vi "Result to Data Warehouse Package.vi"(6 "File Data Objs":T1[](array[typedef]), 7 "Temp Folder":path, 8 "error in":errorcluster, 9 "Test Result":T2={"#attributes"={"Version"="MTE_1.0.0"}, "Station"={"Name"="", "PN"="", "SN"="", "Rev"="", "PC Name"="", "Location"="", "HW_Config"={"HW_Item"=[]}, "SW_Config"={"SW_Item"=[]}}, "Test Run"={"Operator"="", "Start Time"=timestamp(0 s since 1904-01-01), "Duration(s)"=0.0, "Mode"="", "Comment"="", "ProcessStep"=""}, "Test Sequence"={"Name"="", "Config"={"Config_Item"=[]}}, "UUTs"={"UUT"=[]}} {"UUTs"."UUT"."Measurements"."Measurement"."Status" items=["LOG", "PASS", "FAIL", "ERROR"]}, 10 "File Name":string, 11 "Folder":path) -> (0 "error out":errorcluster)   [LabVIEW 2018]
uses:
  TestResult.FullResultData.ctl
  TestResult.Station Info.ctl
  TestResult.HW Item.ctl
  TestResult.SW Item.ctl
  TestResult.Test Run Info.ctl
  TestResult.Test Info.ctl
  TestResult.UUT Result.ctl
  TestResult.Symptom.ctl
  TestResult.Symptom.State.ctl
  Result.Measurement Item.ctl
  Result.Measurement and Attribute Item Status.ctl
  TestResult.UUTInfo.ctl
  Reports/Report.Result FileDataObject.ctl
  <vilib>/KATE/Files/File Utils.lvlib
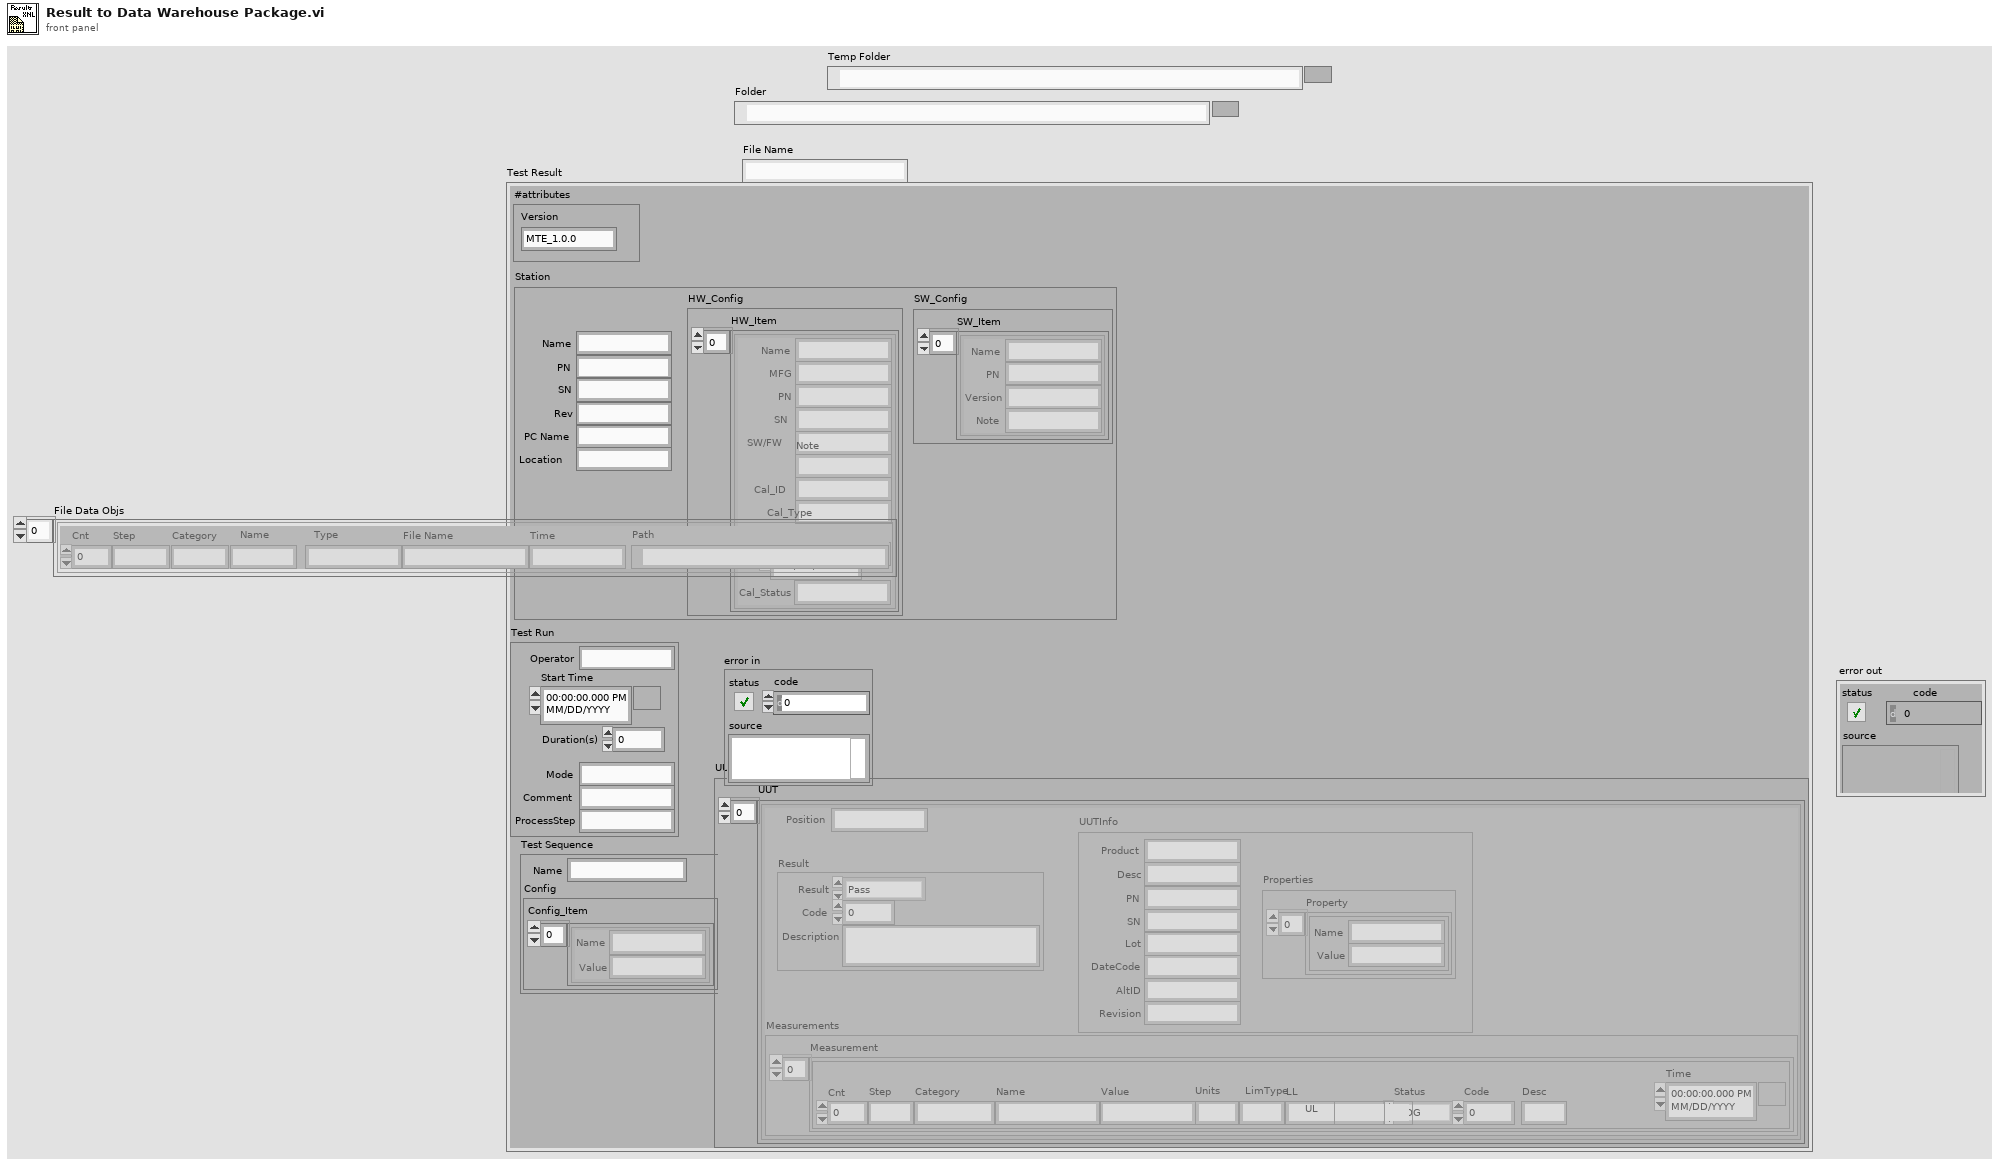
[diagram p1: front panel]
types:
  T1 = typedef "Report.Result FileDataObject.ctl" = cluster{"Cnt":i32, "Step":string, "Category":string, "Name":string, "Type":string, "File Name":string, "Time":string, "Path":path}
  T2 = typedef "TestResult.FullResultData.ctl" = cluster{"#attributes":cluster{"Version":string}, "Station":T3, "Test Run":T6, "Test Sequence":T7, "UUTs":cluster{"UUT":T8[]}}
  T3 = typedef "TestResult.Station Info.ctl" = cluster{"Name":string, "PN":string, "SN":string, "Rev":string, "PC Name":string, "Location":string, "HW_Config":cluster{"HW_Item":T4[]}, "SW_Config":cluster{"SW_Item":T5[]}}
  T4 = typedef "TestResult.HW Item.ctl" = cluster{"Name":string, "MFG":string, "PN":string, "SN":string, "SW/FW":string, "Note":string, "Cal_ID":string, "Cal_Type":string, "Cal_Due_Date":timestamp, "Cal_Status":string}
  T5 = typedef "TestResult.SW Item.ctl" = cluster{"Name":string, "PN":string, "Version":string, "Note":string}
  T6 = typedef "TestResult.Test Run Info.ctl" = cluster{"Operator":string, "Start Time":timestamp, "Duration(s)":dbl, "Mode":string, "Comment":string, "ProcessStep":string}
  T7 = typedef "TestResult.Test Info.ctl" = cluster{"Name":string, "Config":cluster{"Config_Item":cluster{"Name":string, "Value":string}[]}}
  T8 = typedef "TestResult.UUT Result.ctl" = cluster{"Position":string, "Result":T9, "Measurements":cluster{"Measurement":T11[]}, "UUTInfo":T13}
  T9 = typedef "TestResult.Symptom.ctl" = cluster{"Result":T10, "Code":i32, "Description":string}
  T10 = typedef "TestResult.Symptom.State.ctl" = enum16{"Pass", "Fail", "Error", "Aborted", "Completed", "Logged"}
  T11 = typedef "Result.Measurement Item.ctl" = cluster{"Cnt":i32, "Step":string, "Category":string, "Name":string, "Value":string, "Units":string, "LimType":string, "LL":string, "UL":string, "Status":T12, "Code":i32, "Desc":string, "Time":timestamp}
  T12 = typedef "Result.Measurement and Attribute Item Status.ctl" = i32
  T13 = typedef "TestResult.UUTInfo.ctl" = cluster{"Product":string, "Desc":string, "PN":string, "SN":string, "Lot":string, "DateCode":string, "AltID":string, "Revision":string, "Properties":cluster{"Property":cluster{"Name":string, "Value":string}[]}}
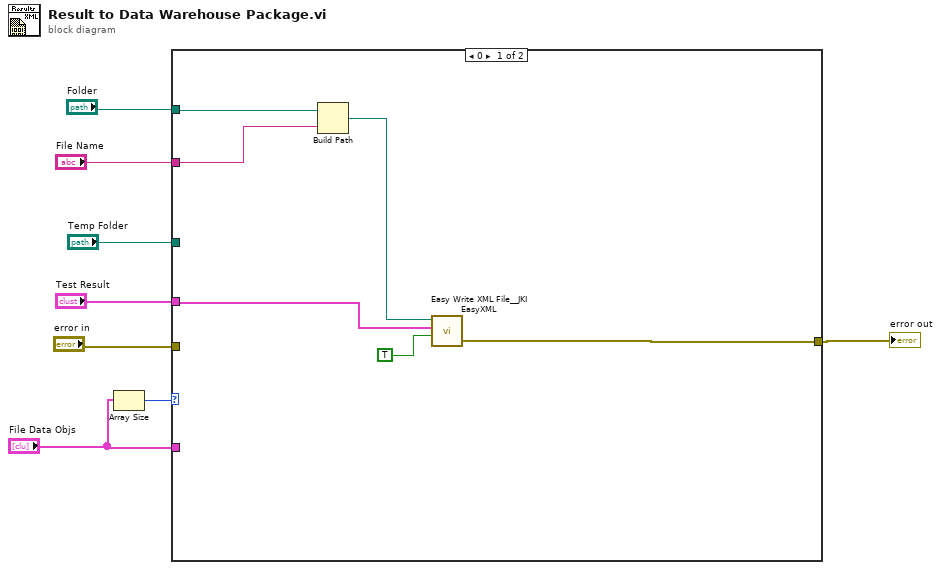
[diagram p0: block diagram]
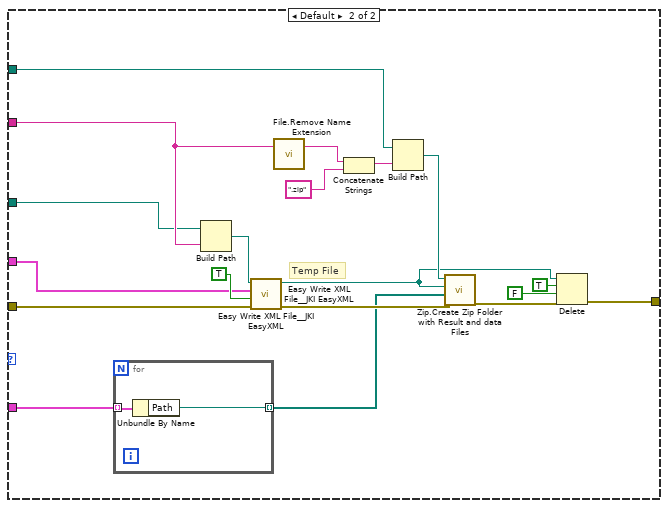
[diagram p2: hidden frame]
diagram:
  n1 = Array Size(array="File Data Objs") -> (size(s)=w2:i32)
  n2 = case shown="0" w2 {
    tunnel: "Test Result" -> [w12 w18]
    tunnel: "error in" -> [_ w33]
    tunnel: "File Data Objs" -> [_ w16]
    tunnel: "File Name" -> [w13 w30]
    tunnel: "Folder" -> [w14 w27]
    tunnel: [w10 w23] -> w4
    tunnel: "Temp Folder" -> [_ w17]
    frame 0 {
      n3 = Build Path(base path=w14, name or relative path=w13) -> (appended path=w11:path)
      n4 = call <vilib>:"Easy Write XML File__JKI EasyXML.vi"("Overwrite File? (false)"=TRUE ("Standalone? (true)"), "LabVIEW Data"=w12, "XML File Path"=w11) -> ("error out"=w10:errorcluster)  [unwired: 7 in, 1 out]
    }
    frame Default {
      # "Temp File"
      n5 = for {
        tunnel: w16 -> [w36] mode=indexing
        tunnel: [w35] -> w15 mode=indexing
        n6 = Unbundle By Name(w36) -> ("Path"=w35:path)
      }
      n7 = Build Path(base path=w17, name or relative path=w30) -> (appended path=w19:path)
      n8 = call <vilib>:"Easy Write XML File__JKI EasyXML.vi"("Overwrite File? (false)"=TRUE, "LabVIEW Data"=w18, "XML File Path"=w19) -> ()  [unwired: 7 in, 2 out]
      n9 = call <vilib>:"Easy Write XML File__JKI EasyXML.vi"("error in (no error)"=w33, "Overwrite File? (false)"=TRUE, "LabVIEW Data"=w18, "XML File Path"=w19) -> ("error out"=w29:errorcluster, "XML File Path (duplicate)"=w24:path)  [unwired: 6 in]
      n10 = call <vilib>:"File.Remove Name Extension.vi"("File Name"=w30) -> ("Name Less Ext"=w32:string)  [unwired: 1 in, 1 out]
      n11 = Concatenate Strings(w32, ".zip" ("string")) -> (w28:string)
      n12 = Build Path(base path=w27, name or relative path=w28) -> (appended path=w26:path)
      n13 = call "Zip.Create Zip Folder with Result and data Files.vi"("error in"=w29, "Data Files"=w15, "Result File"=w24, "Output Zip File"=w26) -> ("error out"=w25:errorcluster)  [unwired: 7 in]
      n14 = Delete(path (use dialog)=w24, entire hierarchy (F)=TRUE, confirm (F)=FALSE, error in=w25) -> (error out=w23:errorcluster)  [unwired: 1 in, 2 out]
    }
  }
  "error out" <- w4
